vi "loadSubVI.vi"(3 "错误输入（无错误）":errorcluster, 4 "VI名称":string, 5 "基路径":path) -> (0 "错误输出":errorcluster, 1 "SubVIRef":refnum<vi>)   [LabVIEW 2018]
panel:
  out "添加的路径":path
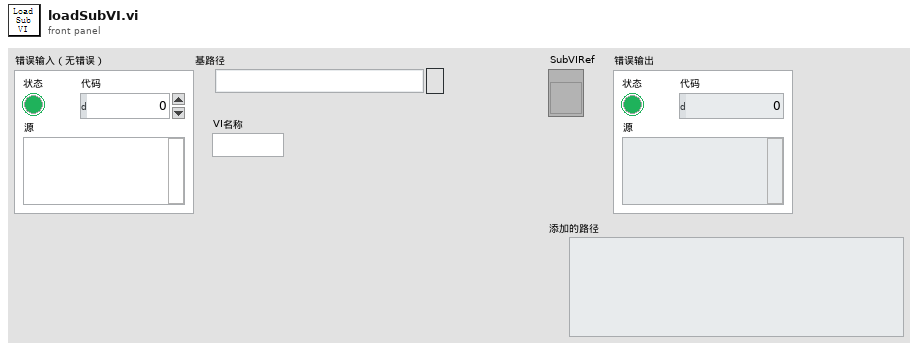
[diagram p1: front panel]
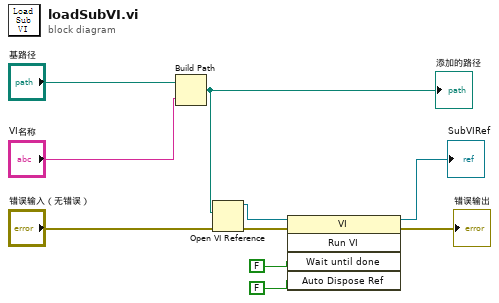
[diagram p0: block diagram]
diagram:
  n1 = Build Path(base path="基路径", name or relative path="VI名称") -> (appended path=w7:path)
  "添加的路径" <- w7
  n2 = Open VI Reference(vi path=w7, error in (no error)="错误输入（无错误）") -> (vi reference=w6:refnum<vi>, error out=w8:errorcluster)  [unwired: 4 in]
  n3 = invoke on="Invoke Node" class="VI" method="Run VI"(reference=w6, error in=w8, "Wait until done"=FALSE ("Wait Until Done"), "Auto Dispose Ref"=FALSE ("Auto Dispose Reference")) -> (reference out=→"SubVIRef":refnum<vi>, error out=→"错误输出":errorcluster)  [unwired: 1 in, 3 out]
